vi "Wrap Data for Measurement Logic Initialization.vi"(11 "measurement configuration":T1 {"SERIAL (SI) CHANNEL" items=["SI0", "SI1"]; "AUTO. VISION DEVICE" items=["PXI1Slot2", "PXI1Slot5"]; "ALGORITHM" items=["BILINEAR", "VNG"]; "PATTERN" items=["GB", "GR", "BG", "RG"]; "INTERPRETATION" items=["Grayscale", "Bayer", "RGB", "YUV422", "YUV420", "Legacy YUV420"]; "SI ACTIVE LANE CNT" items=["1 LANE"=1, "2 LANE"=2, "4 LANE"=4]; "CSI-2 DATA SOURCE" items=["CORRECTED", "RAW"]; "POC SOURCE" items=["NONE", "INTERNAL", "AUXILIARY"]; "REF. CLOCK  (Hz)" format="%#_6p"}) -> (0 "REF. CLOCK  (Hz)":dbl, 1 "RIO HANDLER":string, 2 "CSI-2 DATA SOURCE":u32, 3 "Serial Input Configuration":T2[](array[typedef]) {"RAW Display Parameters"."Bayer Parameters"."Blue Gain" min=0.0 max=3.99 step=0.1 format="%_4g"; "RAW Display Parameters"."Bayer Parameters"."Green Gain" min=0.0 max=3.99 step=0.1 format="%_4g"; "RAW Display Parameters"."Bayer Parameters"."Red Gain" min=0.0 max=3.99 step=0.1 format="%_4g"; "RAW Display Parameters"."Bayer Parameters"."Algorithm" items=["Bilinear", "VNG"]; "RAW Display Parameters"."Bayer Parameters"."Pattern" items=["GB", "GR", "BG", "RG"]}, 4 "POC SOURCE":u32, 5 "appended path":path, 6 "SI ACTIVE LANE CNT":u32, 7 "PATH TO CONFIGURATION SCRIPT":string)   [LabVIEW 2025, in "Automotive Vision.lvclass"]
uses:
  Automotive Vision.lvclass
  Program Files/NI/LVAddons/flexrioii/1/ProjectTemplates/Source/FlexRIO/NI148X/Getting Started/Host/Common/Types/Serial Channel Configuration.ctl
  <instrlib>/FlexRIO/CSI-2/v2/FPGA/Types/Display Parameters.ctl
  <instrlib>/FlexRIO/CSI-2/v2/Common/Types/LLP Data Type.ctl
  Program Files/NI/LVAddons/flexrioii/1/ProjectTemplates/Source/FlexRIO/NI148X/Getting Started/Host/Common/Types/RAW Interpretation for Display.ctl
  Measurement Configuration.ctl
  Automotive Vision.lvclass/Automotive Vision.ctl
  <instrlib>/FlexRIO/CSI-2/v2/Common/NI CSI-2 API Common v2.lvlib
  <instrlib>/FlexRIO/CSI-2/v2/FPGA/NI CSI-2 API FPGA v2.lvlib
  Program Files/NI/LVAddons/flexrioii/1/ProjectTemplates/Source/FlexRIO/NI148X/Getting Started/Host/Common/GettingStarted_Common_148X_Host.lvlib
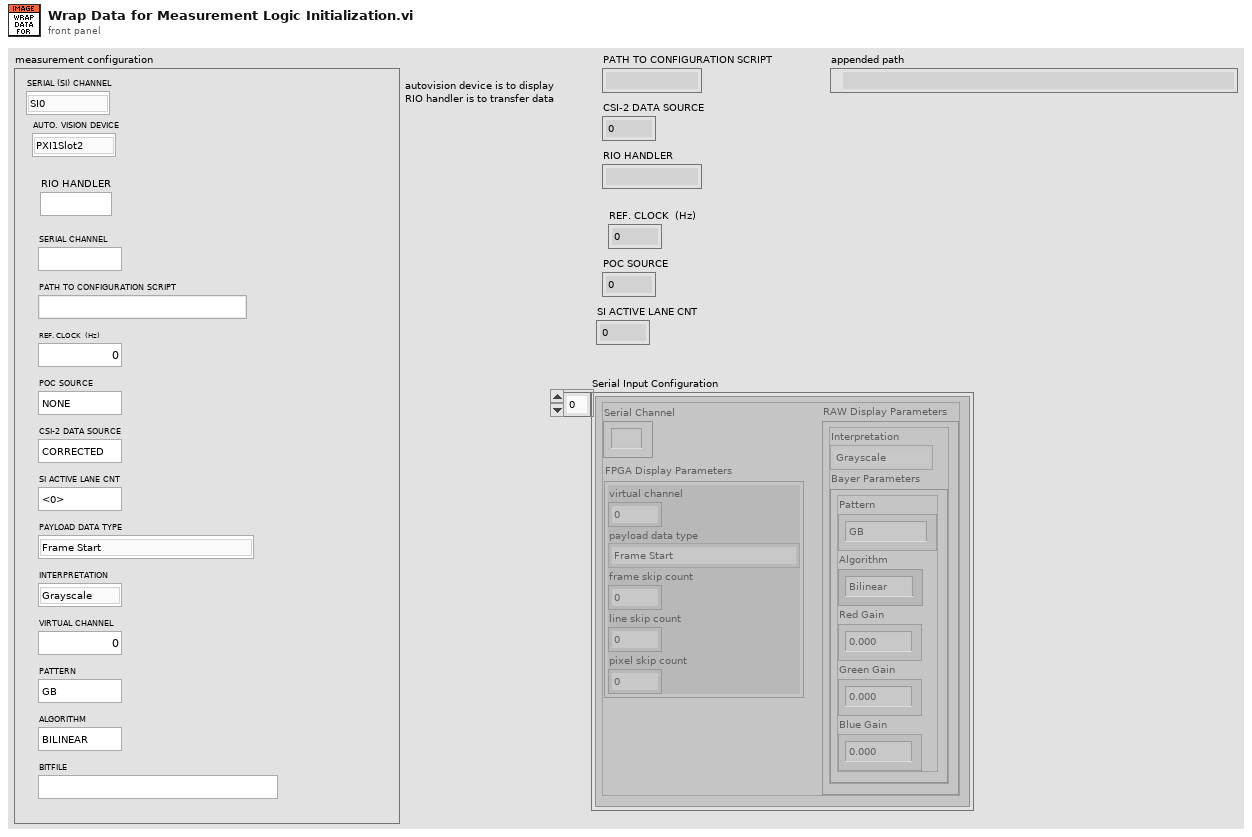
[diagram p1: front panel]
types:
  T1 = typedef "Automotive Vision.lvclass/Measurement Configuration.ctl" = cluster{"SERIAL CHANNEL":string, "PATH TO CONFIGURATION SCRIPT":string, "REF. CLOCK  (Hz)":dbl, "POC SOURCE":u32, "CSI-2 DATA SOURCE":u32, "SI ACTIVE LANE CNT":u32, "PAYLOAD DATA TYPE":enum32{"Frame Start", "Frame End", "Line Start", "Line End", "End of Transmission", "Reserved 0", "Reserved 1", "Reserved 2", "Generic Short Packet 1", "Generic Short Packet 2", "Generic Short Packet 3", "Generic Short Packet 4", "Generic Short Packet 5", "Generic Short Packet 6", "Generic Short Packet 7", "Generic Short Packet 8", "Null", "Blanking Data", "Embedded 8-bit non Image Data", "Generic Long Packet 1", "Generic Long Packet 2", "Generic Long Packet 3", "Generic Long Packet 4", "Reserved 3", "YUV420 8-bit", "YUV420 10-bit", "Legacy YUV420 8-bit", "Reserved 4", "YUV420 8-bit Chroma Shifted", "YUV420 10-bit Chroma Shifted", "YUV422 8-bit", "YUV422 10-bit", "RGB444", "RGB555", "RGB565", "RGB666", "RGB888", "Reserved 5", "Reserved 6", "RAW 24", "RAW 6", "RAW 7", "RAW 8", "RAW 10", "RAW 12", "RAW 14", "RAW 16", "RAW 20", "User Defined 8-bit Data 1", "User Defined 8-bit Data 2", "User Defined 8-bit Data 3", "User Defined 8-bit Data 4", "User Defined 8-bit Data 5", "User Defined 8-bit Data 6", "User Defined 8-bit Data 7", "User Defined 8-bit Data 8", "USL Command", "Reserved 7", "Reserved 8", "Reserved 9", "Reserved 10", "Reserved 11", "Reserved 12", "LRTE EPD Spacer"}, "INTERPRETATION":u32, "VIRTUAL CHANNEL":u32, "PATTERN":u32, "ALGORITHM":u32, "RIO HANDLER":string, "AUTO. VISION DEVICE":u32, "SERIAL (SI) CHANNEL":u32, "BITFILE":string}
  T2 = typedef "GettingStarted_Common_148X_Host.lvlib/Serial Channel Configuration.ctl" = cluster{"Serial Channel":string, "FPGA Display Parameters":T3, "RAW Display Parameters":cluster{"Interpretation":T5, "Bayer Parameters":cluster{"Pattern":i32, "Algorithm":i32, "Red Gain":dbl, "Green Gain":dbl, "Blue Gain":dbl}}}
  T3 = typedef "NI CSI-2 API FPGA v2.lvlib/Display Parameters.ctl" = cluster{"virtual channel":fxp<+,4,4>, "payload data type":T4, "frame skip count":u16, "line skip count":u8, "pixel skip count":fxp<+,5,5>}
  T4 = typedef "NI CSI-2 API Common v2.lvlib/LLP Data Type.ctl" = enum8{"Frame Start", "Frame End", "Line Start", "Line End", "End of Transmission", "Reserved 0", "Reserved 1", "Reserved 2", "Generic Short Packet 1", "Generic Short Packet 2", "Generic Short Packet 3", "Generic Short Packet 4", "Generic Short Packet 5", "Generic Short Packet 6", "Generic Short Packet 7", "Generic Short Packet 8", "Null", "Blanking Data", "Embedded 8-bit non Image Data", "Generic Long Packet 1", "Generic Long Packet 2", "Generic Long Packet 3", "Generic Long Packet 4", "Reserved 3", "YUV420 8-bit", "YUV420 10-bit", "Legacy YUV420 8-bit", "Reserved 4", "YUV420 8-bit Chroma Shifted", "YUV420 10-bit Chroma Shifted", "YUV422 8-bit", "YUV422 10-bit", "RGB444", "RGB555", "RGB565", "RGB666", "RGB888", "Reserved 5", "Reserved 6", "RAW 24", "RAW 6", "RAW 7", "RAW 8", "RAW 10", "RAW 12", "RAW 14", "RAW 16", "RAW 20", "User Defined 8-bit Data 1", "User Defined 8-bit Data 2", "User Defined 8-bit Data 3", "User Defined 8-bit Data 4", "User Defined 8-bit Data 5", "User Defined 8-bit Data 6", "User Defined 8-bit Data 7", "User Defined 8-bit Data 8", "USL Command", "Reserved 7", "Reserved 8", "Reserved 9", "Reserved 10", "Reserved 11", "Reserved 12", "LRTE EPD Spacer"}
  T5 = typedef "GettingStarted_Common_148X_Host.lvlib/RAW Interpretation for Display.ctl" = enum16{"Grayscale", "Bayer", "RGB", "YUV422", "YUV420", "Legacy YUV420"}
  T6 = cluster{"Pattern":i32, "Algorithm":i32, "Red Gain":dbl, "Green Gain":dbl, "Blue Gain":dbl}
  T7 = cluster{"Interpretation":T5, "Bayer Parameters":cluster{"Pattern":i32, "Algorithm":i32, "Red Gain":dbl, "Green Gain":dbl, "Blue Gain":dbl}}
  T8 = enum32{"Frame Start", "Frame End", "Line Start", "Line End", "End of Transmission", "Reserved 0", "Reserved 1", "Reserved 2", "Generic Short Packet 1", "Generic Short Packet 2", "Generic Short Packet 3", "Generic Short Packet 4", "Generic Short Packet 5", "Generic Short Packet 6", "Generic Short Packet 7", "Generic Short Packet 8", "Null", "Blanking Data", "Embedded 8-bit non Image Data", "Generic Long Packet 1", "Generic Long Packet 2", "Generic Long Packet 3", "Generic Long Packet 4", "Reserved 3", "YUV420 8-bit", "YUV420 10-bit", "Legacy YUV420 8-bit", "Reserved 4", "YUV420 8-bit Chroma Shifted", "YUV420 10-bit Chroma Shifted", "YUV422 8-bit", "YUV422 10-bit", "RGB444", "RGB555", "RGB565", "RGB666", "RGB888", "Reserved 5", "Reserved 6", "RAW 24", "RAW 6", "RAW 7", "RAW 8", "RAW 10", "RAW 12", "RAW 14", "RAW 16", "RAW 20", "User Defined 8-bit Data 1", "User Defined 8-bit Data 2", "User Defined 8-bit Data 3", "User Defined 8-bit Data 4", "User Defined 8-bit Data 5", "User Defined 8-bit Data 6", "User Defined 8-bit Data 7", "User Defined 8-bit Data 8", "USL Command", "Reserved 7", "Reserved 8", "Reserved 9", "Reserved 10", "Reserved 11", "Reserved 12", "LRTE EPD Spacer"}
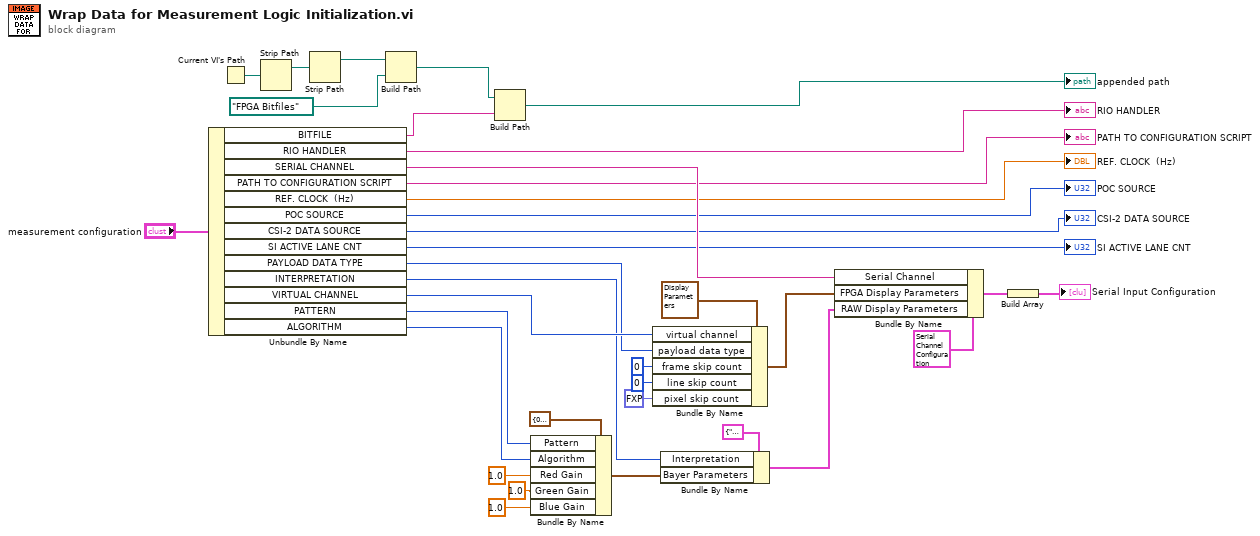
[diagram p0: block diagram]
diagram:
  n1 = Unbundle By Name("measurement configuration") -> ("BITFILE"=w33:string, "RIO HANDLER"=→"RIO HANDLER":string, "SERIAL CHANNEL"=w35:string, "PATH TO CONFIGURATION SCRIPT"=→"PATH TO CONFIGURATION SCRIPT":string, "REF. CLOCK  (Hz)"=→"REF. CLOCK  (Hz)":dbl, "POC SOURCE"=→"POC SOURCE":u32, "CSI-2 DATA SOURCE"=→"CSI-2 DATA SOURCE":u32, "SI ACTIVE LANE CNT"=→"SI ACTIVE LANE CNT":u32, "PAYLOAD DATA TYPE"=w14:T8, "INTERPRETATION"=w17:u32, "VIRTUAL CHANNEL"=w20:u32, "PATTERN"=w19:u32, "ALGORITHM"=w21:u32)
  n2 = Current VI's Path() -> (path=w2:path)
  n3 = Strip Path(path=w2) -> (stripped path=w1:path)  [unwired: 1 out]
  n4 = Strip Path(path=w1) -> (stripped path=w32:path)  [unwired: 1 out]
  n5 = Build Path(base path=w32, name or relative path=path "FPGA Bitfiles" ("base path")) -> (appended path=w31:path)
  n6 = Build Path(base path=w31, name or relative path=w33) -> (appended path=→"appended path":path)
  n7 = Bundle By Name(cluster=T6 {"Pattern"=0, "Algorithm"=0, "Red Gain"=0.0, "Green Gain"=0.0, "Blue Gain"=0.0} ("Bayer Parameters"), "Pattern"=w19, "Algorithm"=w21, "Red Gain"=1.0, "Green Gain"=1.0, "Blue Gain"=1.0) -> (w18:T6)
  n8 = Bundle By Name(cluster=T3 {"virtual channel"=0.0, "payload data type"=enum."Frame Start", "frame skip count"=0, "line skip count"=0, "pixel skip count"=0.0} ("FPGA Display Parameters"), "virtual channel"=w20, "payload data type"=w14, "frame skip count"=u16 0, "line skip count"=u8 0, "pixel skip count"=fxp<+,5,5> 0.0) -> (w13:T3)
  n9 = Bundle By Name(cluster=T7 {"Interpretation"=enum."Grayscale", "Bayer Parameters"={"Pattern"=0, "Algorithm"=0, "Red Gain"=0.0, "Green Gain"=0.0, "Blue Gain"=0.0}} ("RAW Display Parameters"), "Interpretation"=w17, "Bayer Parameters"=w18) -> (w25:T7)
  n10 = Bundle By Name(cluster=T2 {"Serial Channel"="SI0", "FPGA Display Parameters"={"virtual channel"=0.0, "payload data type"=enum."RAW 12", "frame skip count"=0, "line skip count"=0, "pixel skip count"=0.0}, "RAW Display Parameters"={"Interpretation"=enum."Bayer", "Bayer Parameters"={"Pattern"=3, "Algorithm"=0, "Red Gain"=1.0, "Green Gain"=1.0, "Blue Gain"=1.0}}} ("Channel Configurations element"), "Serial Channel"=w35, "FPGA Display Parameters"=w13, "RAW Display Parameters"=w25) -> (w26:T2)
  n11 = Build Array(w26) -> (→"Serial Input Configuration":T2[])
